vi "Network Ping.vi"() -> ()   [LabVIEW 2010]
panel:
  in  "stop":bool
  out "error out":errorcluster
  out "standard output":string
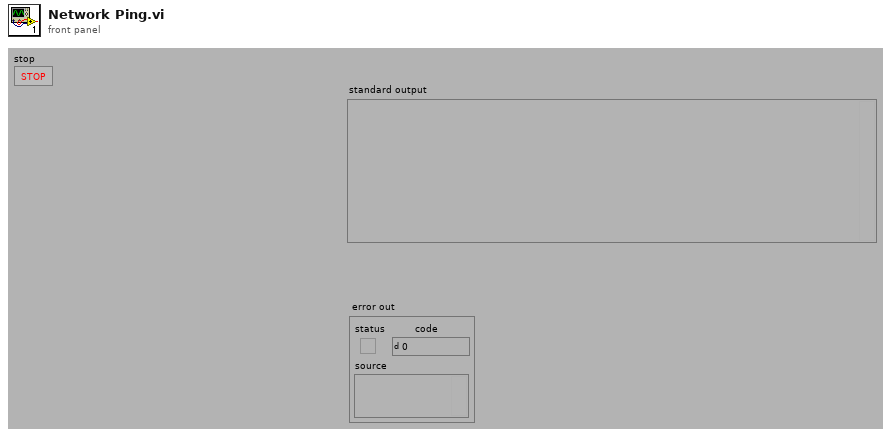
[diagram p1: front panel]
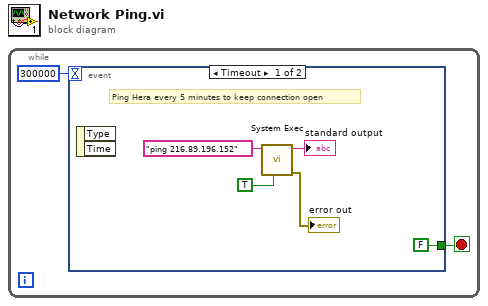
[diagram p0: block diagram]
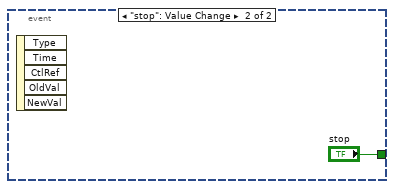
[diagram p2: hidden frame]
diagram:
  n1 = while {
    stop <- w2 stop-if-true
    n2 = event shown="[0] Timeout" {
      selector: _ -> [_ _]
      dyn-events: _ -> [_ _]
      timeout: 300000 -> [_ _]
      tunnel: [FALSE ("stop") "stop"] -> w2
      event Timeout {
        # "Ping Hera every 5 minutes to keep connection open"
        n3 = event-data() -> ()  [unwired: 1 in, 2 out]
        n4 = call <vilib>:"System Exec.vi"("run minimized? (F)"=TRUE, "command line"="ping 216.89.196.152") -> ("error out"=→"error out":errorcluster, "standard output"=→"standard output":string)  [unwired: 6 in, 2 out]
      }
      event "stop": Value Change {
        n5 = event-data() -> ()  [unwired: 1 in, 5 out]
      }
    }
  }
